vi "HoldAndPress.vi"(10 "Holdtime":dbl(slide) min=0.0 max=5.0 scale=0.0..5.0, 11 "Input":bool) -> (0 "Press?":bool, 1 "Long Press":bool, 2 "Quick Press":bool, 3 "Waveform Chart 2":i16(graph), 4 "Waveform Chart":i16(graph), 6 "?":u32)   [LabVIEW 2018]
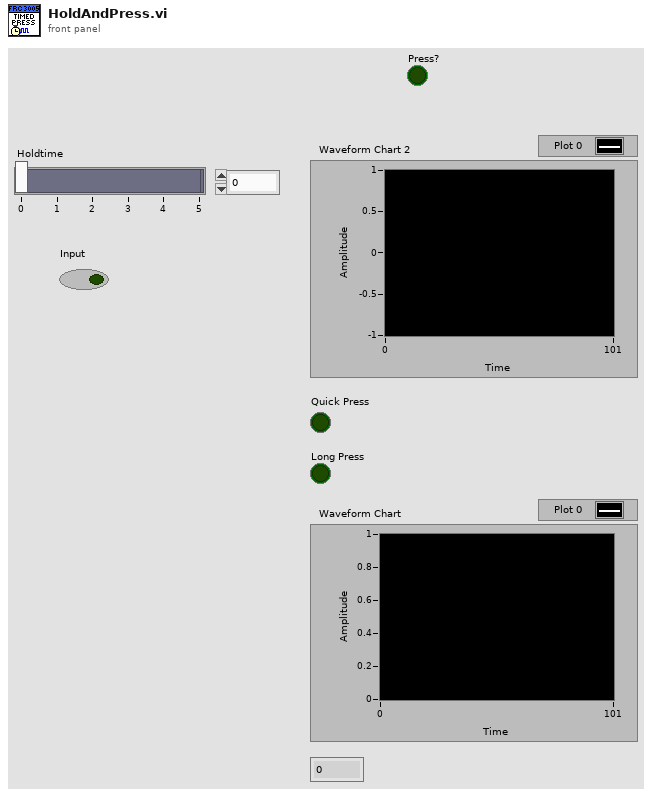
[diagram p1: front panel]
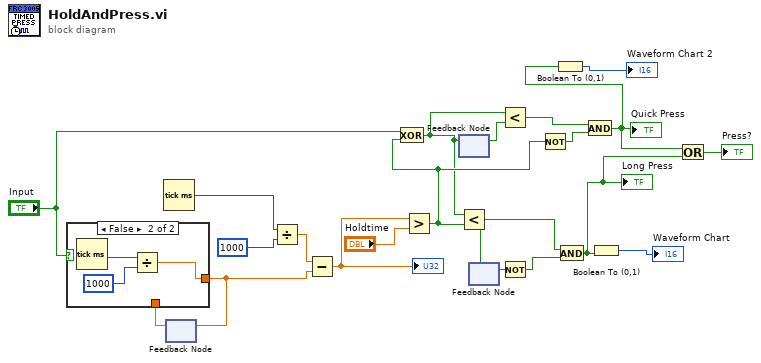
[diagram p0: block diagram]
diagram:
  n1 = Tick Count (ms)() -> (millisecond timer value=w8:u32)
  n2 = feedback #1() -> (w5:dbl)  [unwired: 1 in]
  n3 = case shown="False" "Input" {
    tunnel: [w22 w23] -> w6
    tunnel: w5 -> [w22 _]
    frame True {
    }
    frame False {
      n4 = Tick Count (ms)() -> (millisecond timer value=w25:u32)
      n5 = Divide(x=w25, y=u32 1000) -> (x/y=w23:dbl)
    }
  }
  n6 = feedback-in #1(w6) -> ()
  n7 = Divide(x=w8, y=u32 1000) -> (x/y=w10:dbl)
  n8 = Subtract(x=w10, y=w6) -> (x-y=w7:dbl)
  "?" <- w7
  n9 = Greater?(x=w7, y="Holdtime") -> (0:w21:bool)
  n10 = Exclusive Or(1:w21, 2:"Input") -> (0:w18:bool)
  n11 = feedback #2() -> (w16:bool)  [unwired: 1 in]
  n12 = feedback-in #2(w18) -> ()
  n13 = Less?(x=w18, y=w21) -> (x < y?=w17:bool)
  n14 = feedback #3() -> (w14:bool)  [unwired: 1 in]
  n15 = feedback-in #3(w17) -> ()
  n16 = Less?(x=w18, y=w16) -> (x < y?=w19:bool)
  n17 = Not(x=w14) -> (.not. x?=w15:bool)
  n18 = Not(x=w21) -> (.not. x?=w20:bool)
  n19 = And(x=w17, y=w15) -> (x .and. y?=w3:bool)
  "Long Press" <- w3
  n20 = And(x=w19, y=w20) -> (x .and. y?=w4:bool)
  "Quick Press" <- w4
  n21 = Boolean To (0,1)(Boolean=w4) -> (0, 1=→"Waveform Chart 2":i16)
  n22 = Boolean To (0,1)(Boolean=w3) -> (0, 1=→"Waveform Chart":i16)
  n23 = Or(x=w4, y=w3) -> (x .or. y?=→"Press?":bool)
